vi "stop.vi"(8 "error in (no error)":errorcluster, 10 "stop?":bool, 11 "k3390_AWG in":refnum<class "k3390_AWG.lvclass">) -> (0 "error out":errorcluster, 2 "hasStopped":bool, 3 "k3390_AWG out":refnum<class "k3390_AWG.lvclass">)   [LabVIEW 2011, in "Hardware.lvlib" / "Channels.lvlib" / "k3390_AWG.lvclass"]
uses:
  k3390_AWG.lvclass
  k3390_AWG.lvclass/k3390_AWG.ctl
  <instrlib>/Keithley 3390/Keithley 3390.lvlib
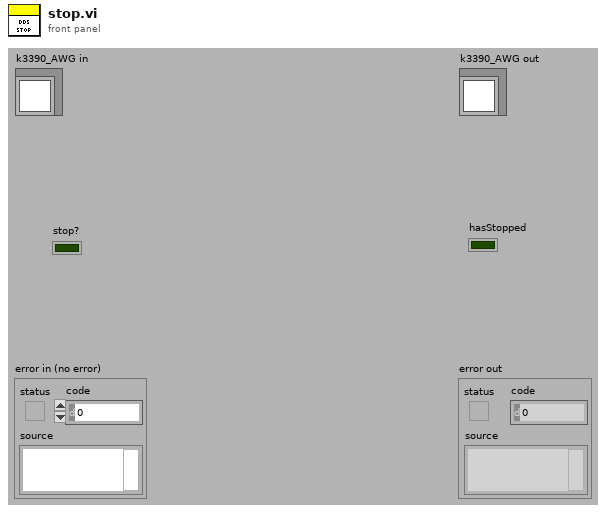
[diagram p1: front panel]
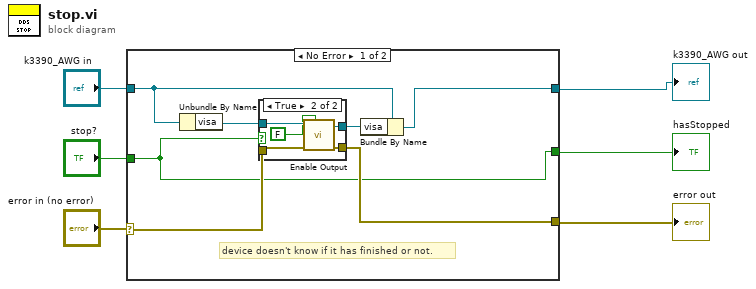
[diagram p0: block diagram]
diagram:
  n1 = case shown="No Error" "error in (no error)" {
    selector: "error in (no error)" -> [w12 w21]
    tunnel: [w8 w23] -> w6
    tunnel: "k3390_AWG in" -> [w9 w23]
    tunnel: [w11 w21] -> w3
    tunnel: "stop?" -> [w7 w22]
    tunnel: [w7 w22] -> w1
    frame No Error {
      # "device doesn't know if it has finished or not."
      n2 = Unbundle By Name(w9) -> ("visa"=w13:refnum<visa-resource-name>)
      n3 = case shown="True" w7 {
        tunnel: w13 -> [w15 w20]
        tunnel: w12 -> [w14 w19]
        tunnel: [w14 w18] -> w11
        tunnel: [w15 w17] -> w10
        frame False {
        }
        frame True {
          n4 = call <instrlib>:"Enable Output.vi"("Enable Output (T: Enable)"=FALSE, "error in (no error)"=w19, "VISA resource name"=w20) -> ("error out"=w18:errorcluster, "VISA resource name out"=w17:refnum<visa-resource-name>)  [unwired: 7 in]
        }
      }
      n5 = Bundle By Name(cluster=w9, "visa"=w10) -> (w8:refnum<class "k3390_AWG.lvclass">)
    }
    frame Error {
    }
  }
  "error out" <- w3
  "k3390_AWG out" <- w6
  "hasStopped" <- w1
